vi "JSON_Read_Multiple_ERDS.vi"(2 "Json File Path":path, 7 "ERD Data Out":cluster{"ERD Number":u16, "Data":string}[](array[cluster]) {"ERD Number" format="%.0x"}, 11 "error in":errorcluster) -> (8 "Array":cluster{"ERD Number":u16, "Data":string}[](array[cluster]), 15 "error out":errorcluster)   [LabVIEW 2021]
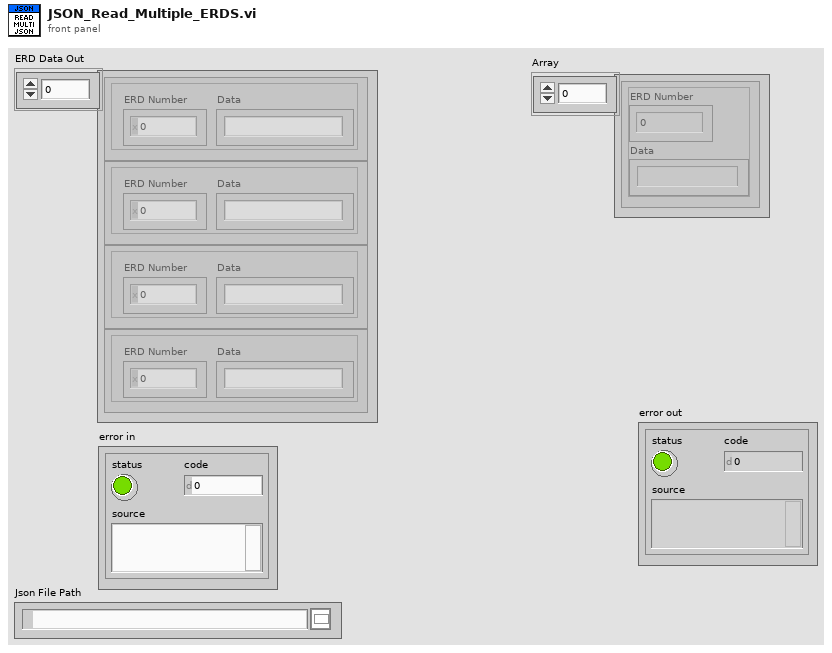
[diagram p1: front panel]
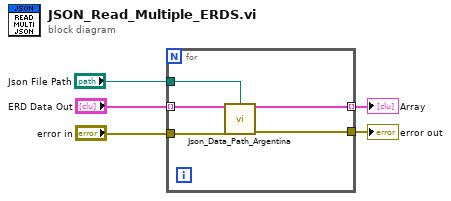
[diagram p0: block diagram]
diagram:
  n1 = for {
    tunnel: "ERD Data Out" -> [w10] mode=indexing
    tunnel: "error in" -> [w9]
    tunnel: [w8] -> w3
    tunnel: [w7] -> w2 mode=indexing
    tunnel: "Json File Path" -> [w6]
    n2 = call "Json_Data_Path_Argentina.vi"("ERD Cluster"=w10, "Json File Path"=w6, "error in"=w9) -> ("ERD JSON"=w7:cluster{"ERD Number":u16, "Data":string}, "error out"=w8:errorcluster)  [unwired: 11 in]
  }
  "error out" <- w3
  "Array" <- w2
